vi "create_save_folder.vi"(0 "Day folder":string, 1 "Measuring number":i32=-1, 2 "Measuring folder":string, 3 "error in":errorcluster caption="Fehler (Eingang, kein Fehler)") -> (7 "Save Folder":string, 10 "Error Out":errorcluster)   [LabVIEW 2009]
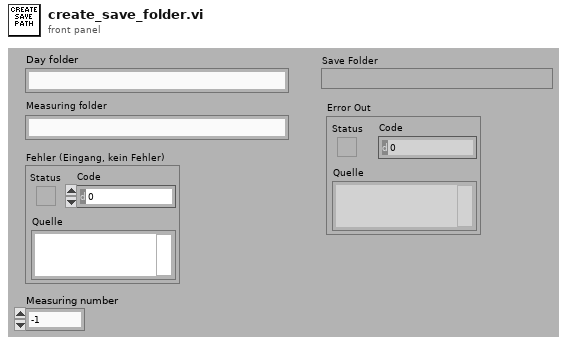
[diagram p1: front panel]
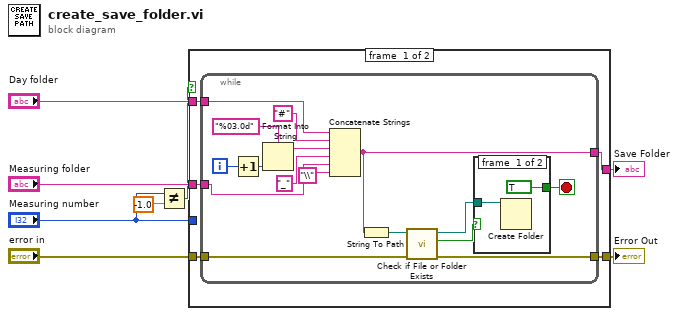
[diagram p0: block diagram]
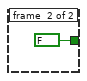
[diagram p2: hidden frame]
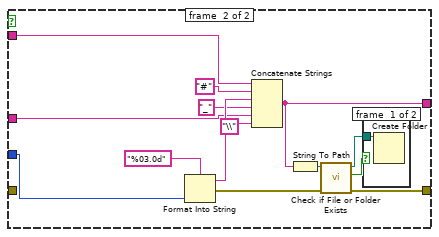
[diagram p3: hidden frame]
diagram:
  n1 = Not Equal?(x="Measuring number", y=-1.0) -> (x != y?=w3:bool)
  n2 = case shown="False" w3 {
    tunnel: "Day folder" -> [w13 w46]
    tunnel: [w12 w39] -> w7
    tunnel: "Measuring folder" -> [w11 w34]
    tunnel: [w10 w38] -> w5
    tunnel: "error in" -> [w9 _]
    tunnel: "Measuring number" -> [_ w42]
    frame #0 {
      n3 = while {
        tunnel: w13 -> [w19]
        tunnel: [w18] -> w12
        tunnel: w11 -> [w14]
        tunnel: [w17] -> w10
        tunnel: w9 -> [w16]
        i -> [w24]
        stop <- w23 stop-if-true
        n4 = Increment(x=w24) -> (x+1=w22:i32)
        n5 = Format Into String(format string="%03.0d" ("Eingangs-String"), w22) -> (resulting string=w21:string)  [unwired: 2 in, 1 out]
        n6 = Concatenate Strings(w19, "#" ("String"), w21, "_" ("String"), w14, "\\" ("String")) -> (w18:string)
        n7 = String To Path(string=w18) -> (path=w29:path)
        n8 = call <vilib>:"Check if File or Folder Exists.vi"("error in (no error)"=w16, "path"=w29) -> ("error out"=w17:errorcluster, "file or folder exists?"=w28:bool, "dup path"=w27:path)  [unwired: 7 in]
        n9 = case shown="False" w28 {
          tunnel: w27 -> [w31 _]
          tunnel: [TRUE FALSE] -> w23
          frame #0 {
            n10 = Create Folder(path (use dialog)=w31) -> ()  [unwired: 2 in, 3 out]
          }
          frame #1 {
          }
        }
      }
    }
    frame #1 {
      n11 = Format Into String(format string="%03.0d" ("Eingangs-String"), w42) -> (resulting string=w35:string, error out=w41:errorcluster)  [unwired: 2 in]
      n12 = Concatenate Strings(w46, "#" ("String"), w35, "_" ("String"), w34, "\\" ("String")) -> (w39:string)
      n13 = String To Path(string=w39) -> (path=w40:path)
      n14 = call <vilib>:"Check if File or Folder Exists.vi"("error in (no error)"=w41, "path"=w40) -> ("error out"=w38:errorcluster, "file or folder exists?"=w37:bool, "dup path"=w36:path)  [unwired: 7 in]
      n15 = case shown="False" w37 {
        tunnel: w36 -> [w47 _]
        frame #0 {
          n16 = Create Folder(path (use dialog)=w47) -> ()  [unwired: 2 in, 3 out]
        }
        frame #1 {
        }
      }
    }
  }
  "Save Folder" <- w7
  "Error Out" <- w5
